vi "Write Configuration File from User.vi"(8 "error in":errorcluster, 10 "Test Configuration":T1) -> (0 "error out":errorcluster, 3 "Cancelled?":bool)   [LabVIEW 2015]
uses:
  Controls/Test Configuration.ctl
  Controls/Test Information.ctl
  Controls/Vacuum Test.ctl
  Controls/Test Timing.ctl
  Controls/Vaccum Thresholds.ctl
  Controls/Helium Test.ctl
  Controls/Helium Thresholds.ctl
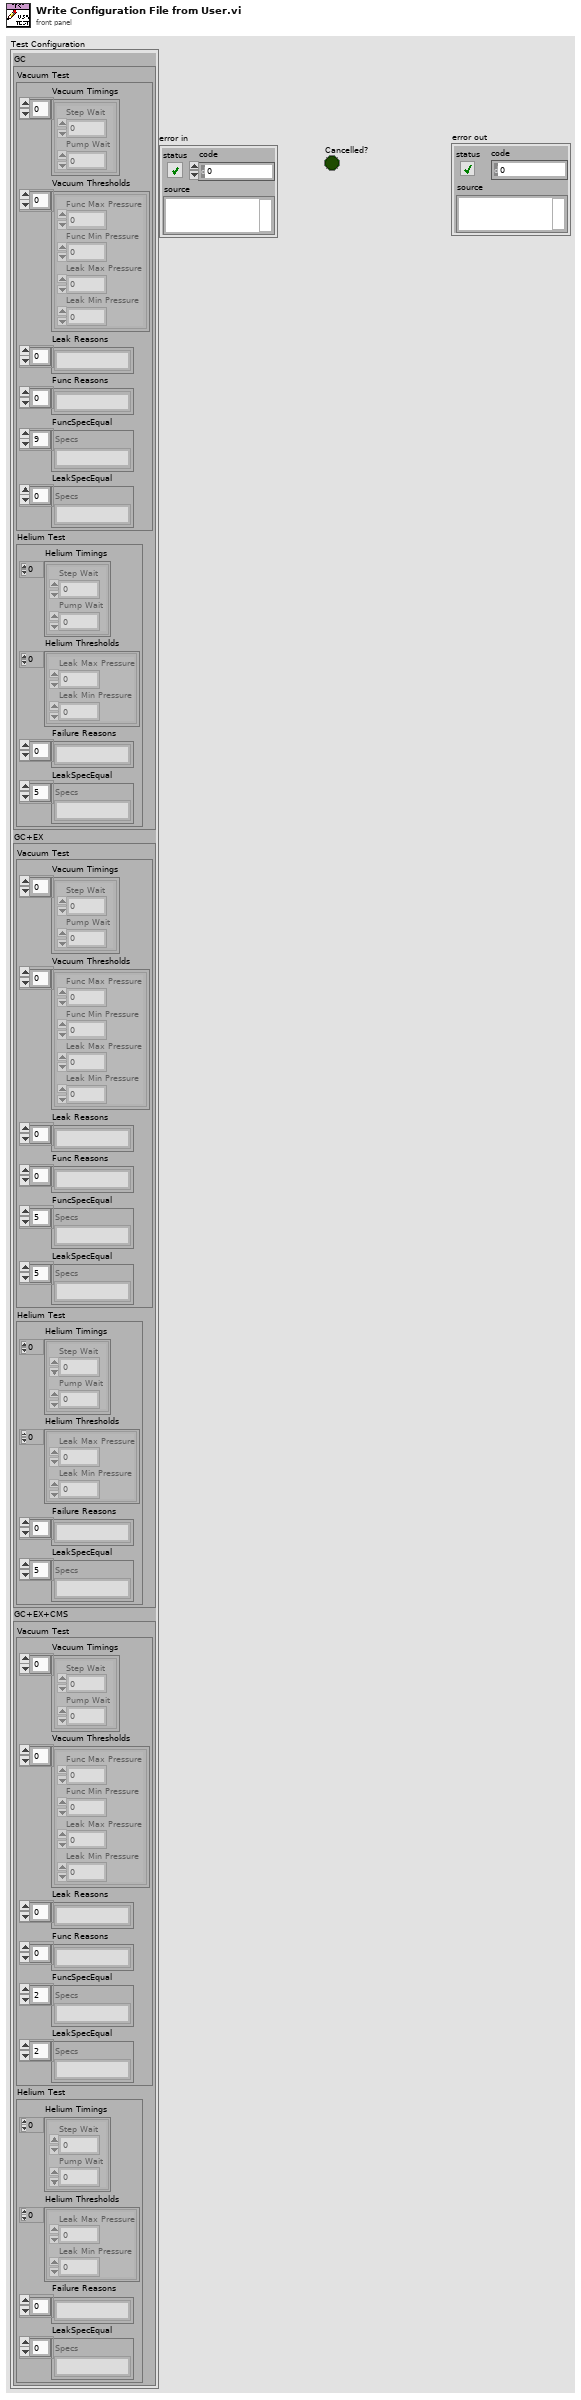
[diagram p1: front panel]
types:
  T1 = typedef "Test Configuration.ctl" = cluster{"GC":T2, "GC+EX":T2, "GC+EX+CMS":T2}
  T2 = typedef "Test Information.ctl" = cluster{"Vacuum Test":T3, "Helium Test":T6}
  T3 = typedef "Vacuum Test.ctl" = cluster{"Vacuum Timings":T4[], "Vacuum Thresholds":T5[], "Leak Reasons":string[], "Func Reasons":string[], "FuncSpecEqual":string[], "LeakSpecEqual":string[]}
  T4 = typedef "Test Timing.ctl" = cluster{"Step Wait":dbl, "Pump Wait":dbl}
  T5 = typedef "Vaccum Thresholds.ctl" = cluster{"Func Max Pressure":dbl, "Func Min Pressure":dbl, "Leak Max Pressure":dbl, "Leak Min Pressure":dbl}
  T6 = typedef "Helium Test.ctl" = cluster{"Helium Timings":T4[], "Helium Thresholds":T7[], "Failure Reasons":string[], "LeakSpecEqual":string[]}
  T7 = typedef "Helium Thresholds.ctl" = cluster{"Leak Max Pressure":dbl, "Leak Min Pressure":dbl}
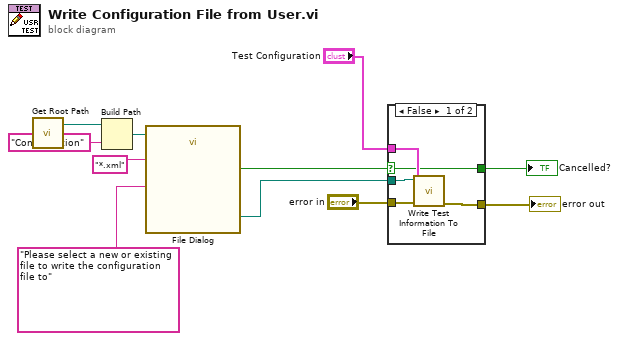
[diagram p0: block diagram]
diagram:
  n1 = call "Get Root Path.vi"() -> ("Root Path"=w1:path)  [unwired: 11 in]
  n2 = Build Path(base path=w1, name or relative path="Configuration") -> (appended path=w10:path)
  n3 = call "File Dialog"("start path"=w10, "prompt"="Please select a new or existing file to write the configuration file to", "pattern (all files)"="*.xml") -> ("selected path"=w6:path, "cancelled"=w4:bool)  [unwired: 9 in, 2 out]
  n4 = case shown="False" w4 {
    selector: w4 -> [w12 w17]
    tunnel: "error in" -> [w16 w18]
    tunnel: [w15 w18] -> w7
    tunnel: w6 -> [w14 _]
    tunnel: "Test Configuration" -> [w13 _]
    tunnel: [w12 w17] -> w3
    frame False {
      n5 = call "Write Test Information To File.vi"("error in"=w16, "Test Configuration"=w13, "base path"=w14) -> ("error out"=w15:errorcluster)  [unwired: 8 in]
    }
    frame True {
    }
  }
  "error out" <- w7
  "Cancelled?" <- w3
